vi "finalise_sweep.vi"(8 "error in (no error)":errorcluster, 11 "ImagingModeMG090624Camera in":refnum<class "ImagingModeMG090624Camera.lvclass">) -> (0 "error out":errorcluster, 3 "ImagingModeMG090624Camera out":refnum<class "ImagingModeMG090624Camera.lvclass">)   [LabVIEW 2010, in "ImagingModeMG090624Camera.lvclass"]
uses:
  ImagingModeMG090624Camera.lvclass
  ImagingModeMG090624Camera.lvclass/ImagingModeMG090624Camera.ctl
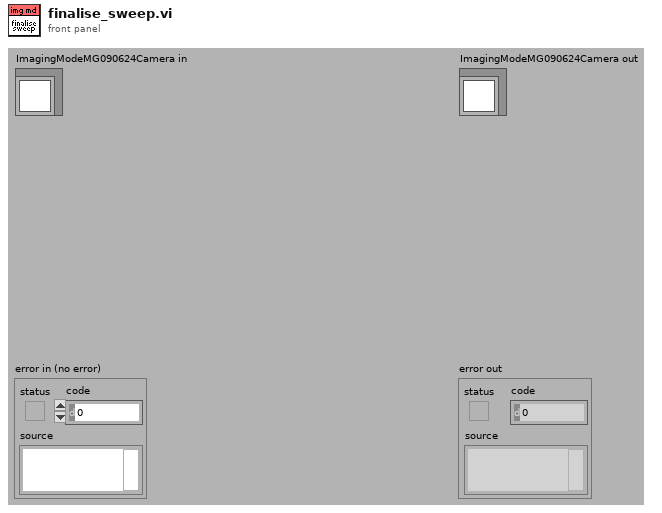
[diagram p1: front panel]
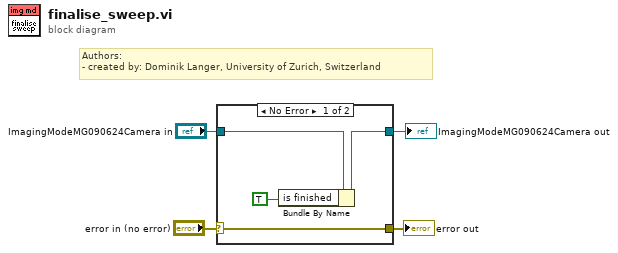
[diagram p0: block diagram]
diagram:
  # "Authors: \n- created by: Dominik Langer, University of Zurich, Switzerland"
  n1 = case shown="No Error" "error in (no error)" {
    selector: "error in (no error)" -> [w8 w10]
    tunnel: [w8 w10] -> w3
    tunnel: [w6 w9] -> w1
    tunnel: "ImagingModeMG090624Camera in" -> [w7 w9]
    frame No Error {
      n2 = Bundle By Name(cluster=w7, "is finished"=TRUE) -> (w6:refnum<class "ImagingModeMG090624Camera.lvclass">)
    }
    frame Error {
    }
  }
  "error out" <- w3
  "ImagingModeMG090624Camera out" <- w1
